vi "Read Ip addr.vi"(8 "error in (no error)":errorcluster, 11 "MBParam in":refnum<class "MBTCP Param.lvclass">) -> (0 "error out":errorcluster, 2 "IP address":T1, 3 "MBParam out":refnum<class "MBTCP Param.lvclass">)   [LabVIEW 2021, in "MBParam.lvlib" / "MBTCP Param.lvclass"]
uses:
  MBTCP Param.lvclass
  MBTCP Param.lvclass/MBTCP Param.ctl
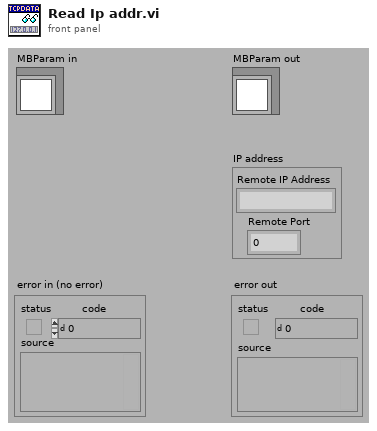
[diagram p1: front panel]
types:
  T1 = cluster{"Remote IP Address":string, "Remote Port":u16}
  T2 = typedef "MBParam.lvlib/MBTCP Param.lvclass/timeouts.ctl" = cluster{"conn_timeout":i32, "reconn_timeout":i32, "N attempt max":i32, "t_reset_TTL":i32, "write_timeout":i32, "read_timeout":i32, "period":i32}
  T3 = cluster{"IP address":cluster{"Remote IP Address":string, "Remote Port":u16}, "timeouts":T2}
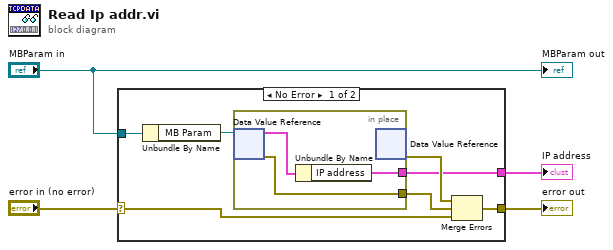
[diagram p0: block diagram]
diagram:
  n1 = case shown="No Error" "error in (no error)" {
    selector: "error in (no error)" -> [w6 w15]
    tunnel: [w10 w15] -> w4
    tunnel: [w5 _] -> w3
    tunnel: "MBParam in" -> [w11 _]
    frame No Error {
      n2 = Unbundle By Name(w11) -> ("MB Param"=w7:refnum<data-value>)
      n3 = in-place {
        in-place-border: [w14] -> w8
        in-place-border: [w12] -> w5
        n4 = in-place-dvr #1(w7) -> (w13:T3, w14:errorcluster)
        n5 = Unbundle By Name(w13) -> ("IP address"=w12:T1)
        n6 = in-place-dvr #1() -> (w9:errorcluster)  [unwired: 1 in, 1 out]
      }
      n7 = Merge Errors(w9, w8, w6) -> (w10:errorcluster)
    }
    frame Error {
    }
  }
  "error out" <- w4
  "IP address" <- w3
  "MBParam out" <- "MBParam in"
